vi "EtherNet CIP WriteTimer_Control_or_Counter_Array.vi"(0 "Connection Cluster":T2={"TCP Connection"=refnum, "Session"=[], "EtherNet/IP Device Address"="172.20.37.243"} {"Session" format="0x%02x"}, 5 "Tag":string, 9 "CONTROL/TIMER/COUNTER":T1, 11 "error in":errorcluster) -> (4 "Connection Cluster Out":T2, 15 "error out":errorcluster)   [LabVIEW 2012]
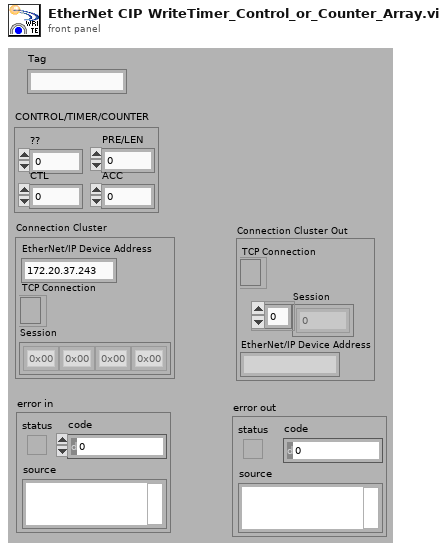
[diagram p1: front panel]
types:
  T1 = cluster{"??":u16, "CTL":u32, "PRE/LEN":u32, "ACC":u32}
  T2 = cluster{"TCP Connection":refnum<k5>, "Session":u8[], "EtherNet/IP Device Address":string}
  T3 = enum16{"No Data", "BOOL", "BIT Array", "SINT", "INT", "DINT", "REAL", "TIMER/CONTROL/COUNTER"}
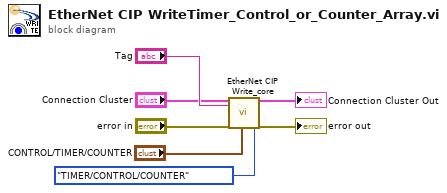
[diagram p0: block diagram]
diagram:
  n1 = call "EtherNet CIP Write_core.vi"("Connection Cluster"="Connection Cluster", "Tag"="Tag", "error in"="error in", "CONTROL/TIMER/COUNTER"="CONTROL/TIMER/COUNTER", "Datatype"=T3."TIMER/CONTROL/COUNTER") -> ("Connection Cluster Out"=→"Connection Cluster Out":T2, "error out"=→"error out":errorcluster)  [unwired: 13 in]
